vi "Lin Daten aufarbeiten.vi"(0 "Eingabetabelle":T4, 1 "Index (Seite)":i32, 3 "Stufen Tabelle":T3, 4 "Zeile":i32, 5 "Lin-Polynom":T5={"Messgerät"="", "Kalibrator (Gasteiler)"="", "Bearbeiter/in"="", "Komponente"="", "Zeitstempel"=timestamp(0 s since 1904-01-01), "F_max gefordert (%)"=0.0, "F_max in %"=0.0, "F_max in ppm"=0.0, "Vorschlag Ordnung"=0, "Polynom OK"=FALSE, "Polynomkoeff."=[], "Prüfgas Konzentration"=0.0, "Pfad EPA"="", "Pfad_LIN"="", "Gasnummer:"=0, "Komponentenauswahl"=[], "Verdünnungsgas"=0, "Zeitdauer Stufe"=0.0, "Anzahl Stufen"=0.0, "F_max in % EPA"=0.0, "F_max in ppm EPA"=0.0, "F_max in % LIN"=0.0, "F_max in ppm LIN"=0.0, "Punkte umkehren"=FALSE, "EPA Optionsfeld"=enum."Rohwert", "Autolin Hovacal"=enum."Optionsauswahl 2", "Spanfactors"=[], "Kalibrierauswahl"=0, "Conditions:"=0, "Gasflaschen Nr.:"="", "Bottle Accuracy"=0.0, "Konfig Gasflasche"=FALSE, "Gasflasche"=0, "HovaCAL Flow AutoLin"={"HovaCAL Flow Input Cluster"=0.0}, "MFC Output"={"Run"=FALSE}, "Gas Ablaufdatum"=timestamp(0 s since 1904-01-01), "Lin Modus"=0, "zusätzliche Zeitdauer Erster Punkt"=0.0, "Offsets"=[]} {"zusätzliche Zeitdauer Erster Punkt" format="%#_5g"; "Lin Modus" items=["Cal Gas to PNS", "Cal Gas to Samplepoint", "Measure"]; "Gas Ablaufdatum" format="%<%d.%m.%Y>T"; "HovaCAL Flow AutoLin"."HovaCAL Flow Input Cluster" format="%.2f"; "Gasflasche" items=["----"=10000, "IAG MG"=0, "IAG NH3 3000"=1, "IAG NH3 2000"=2, "IAG NH3 200"=3]; "Conditions:" items=["field", "laboratory"]; "Kalibrierauswahl" items=["Inaktiv", "Aktiv"]; "Anzahl Stufen" format="%#_5g"; "Zeitdauer Stufe" format="%#_5g"; "Verdünnungsgas" items=["N2", "O2"]; "Komponentenauswahl"."Konzentration" format="%#.6f"; "Gasnummer:" min=1 max=5; "Prüfgas Konzentration" format="%#.6f"; "Polynomkoeff." format="%#_18f"}, 6 "EGAK":string[](array[string]), 7 "error in (no error)":errorcluster caption="Fehler (Eingang, kein Fehler)", 8 "Polynom-Ordnung":i32, 9 "TabellenArray":string[][][](array[string]), 10 "Aktiv":T1, 12 "LINArray":bool[][](array[boolean]), 13 "Aktionen":T19, 14 "EPA Array":bool[][](array[boolean])) -> (16 "Aktiv EPA":T1, 17 "TabellenArray":string[][][](array[string]), 18 "Aktiv LIN":bool[](array[boolean]), 20 "Eingabetabelle":T4, 21 "Index (Seite) out":i32, 22 "Ergebnis Lin":string[][](array[string]), 23 "Stufen Tabelle":T3, 24 "EPA Auswertung":cluster{sgl[], sgl[], bool[]}, 25 "Lin-Polynom":T5={"Messgerät"="", "Kalibrator (Gasteiler)"="", "Bearbeiter/in"="", "Komponente"="", "Zeitstempel"=timestamp(0 s since 1904-01-01), "F_max gefordert (%)"=0.0, "F_max in %"=0.0, "F_max in ppm"=0.0, "Vorschlag Ordnung"=0, "Polynom OK"=FALSE, "Polynomkoeff."=[], "Prüfgas Konzentration"=0.0, "Pfad EPA"="", "Pfad_LIN"="", "Gasnummer:"=0, "Komponentenauswahl"=[], "Verdünnungsgas"=0, "Zeitdauer Stufe"=0.0, "Anzahl Stufen"=0.0, "F_max in % EPA"=0.0, "F_max in ppm EPA"=0.0, "F_max in % LIN"=0.0, "F_max in ppm LIN"=0.0, "Punkte umkehren"=FALSE, "EPA Optionsfeld"=enum."Rohwert", "Autolin Hovacal"=enum."Optionsauswahl 2", "Spanfactors"=[], "Kalibrierauswahl"=0, "Conditions:"=0, "Gasflaschen Nr.:"="", "Bottle Accuracy"=0.0, "Konfig Gasflasche"=FALSE, "Gasflasche"=0, "HovaCAL Flow AutoLin"={"HovaCAL Flow Input Cluster"=0.0}, "MFC Output"={"Run"=FALSE}, "Gas Ablaufdatum"=timestamp(0 s since 1904-01-01), "Lin Modus"=0, "zusätzliche Zeitdauer Erster Punkt"=0.0, "Offsets"=[]} {"zusätzliche Zeitdauer Erster Punkt" format="%#_5g"; "Lin Modus" items=["Cal Gas to PNS", "Cal Gas to Samplepoint", "Measure"]; "Gas Ablaufdatum" format="%<%d.%m.%Y>T"; "HovaCAL Flow AutoLin"."HovaCAL Flow Input Cluster" format="%.2f"; "Gasflasche" items=["----"=10000, "IAG MG"=0, "IAG NH3 3000"=1, "IAG NH3 2000"=2, "IAG NH3 200"=3]; "Conditions:" items=["field", "laboratory"]; "Kalibrierauswahl" items=["Inaktiv", "Aktiv"]; "Anzahl Stufen" format="%#_5g"; "Zeitdauer Stufe" format="%#_5g"; "Verdünnungsgas" items=["N2", "O2"]; "Komponentenauswahl"."Konzentration" format="%#.6f"; "Gasnummer:" min=1 max=5; "Prüfgas Konzentration" format="%#.6f"; "Polynomkoeff." format="%#_18f"}, 26 "EKAG":string[](array[string]), 27 "error out":errorcluster caption="Fehler (Ausgang)")   [LabVIEW 2020, in "Linearisierung v2.lvlib"]
uses:
  Linearisierung v2.lvlib
  Aktion Lin Daten aufarbeiten.ctl
  Lin-Polynom Daten.ctl
  KomponentenArray.ctl
  Visualisierungs Elemente/Auswahlfeld.ctl
  Visualisierungs Elemente/Zahlen-Eingabefeld.ctl
  EPA Optionsfeld.ctl
  Gasteiler/HovaCal/AutoLin Hovacal.ctl
  Kalibrieroption.ctl
  EPA1065-307/Condition.ctl
  Seiten/System Einstellungen V2/Konfig Gasflasche.ctl
  Seiten/System Einstellungen V2/Gasflasche Auswahl.ctl
  Gasteiler/HovaCAL_Interface/Controls/Flow Einstellung.ctl
  Gasteiler/HovaCAL_Interface/Controls/Pump state.ctl
  Seiten/CalGas Aufschaltung/Lin Modus.ctl
  Eingabetabelle.ctl
  Gasteiler/Stufen Tabelle.ctl
  AktivArray.ctl
  AktivButton.ctl
  Sprachverwaltung/FGV Aktion Tabelle zerlegen.ctl
  Allgemein/allgemeine Sub-VIs.lvlib
  EPA1065-307/Linearity verification 1065-307.lvlib
  Sprachverwaltung/Sprachverwaltung.lvlib
  Gasteiler/Gasteiler.lvlib
  Gasteiler/HovaCal/HovaCal.lvlib
  Seiten/System Einstellungen V2/System Einstellungen V2.lvlib
  Gasteiler/HovaCAL_Interface/Controls/Controls.lvlib
  Seiten/CalGas Aufschaltung/CalGas Aufschaltung.lvlib
panel:
  # "Tabelle:\n0.....Sollwert\n1.....Istwert\n2.....Rohwert\n3.....linearisiert\n4.....abs.Fehler ppm\n5.....Fehler in %\n6.....Deviation\n7.....Temp.Messzelle\n8.....Druck Messzelle\n9.....abs.Fehler ppm linearisiert\n10....Fehler in % linearisiert\n11....abs.Fehler ppm EPA\n12....Fehler in % EPA\n13....abs.Fehler ppm Rohwert\n14....Fehler in % Rohwert"
  # "%"
  # "%"
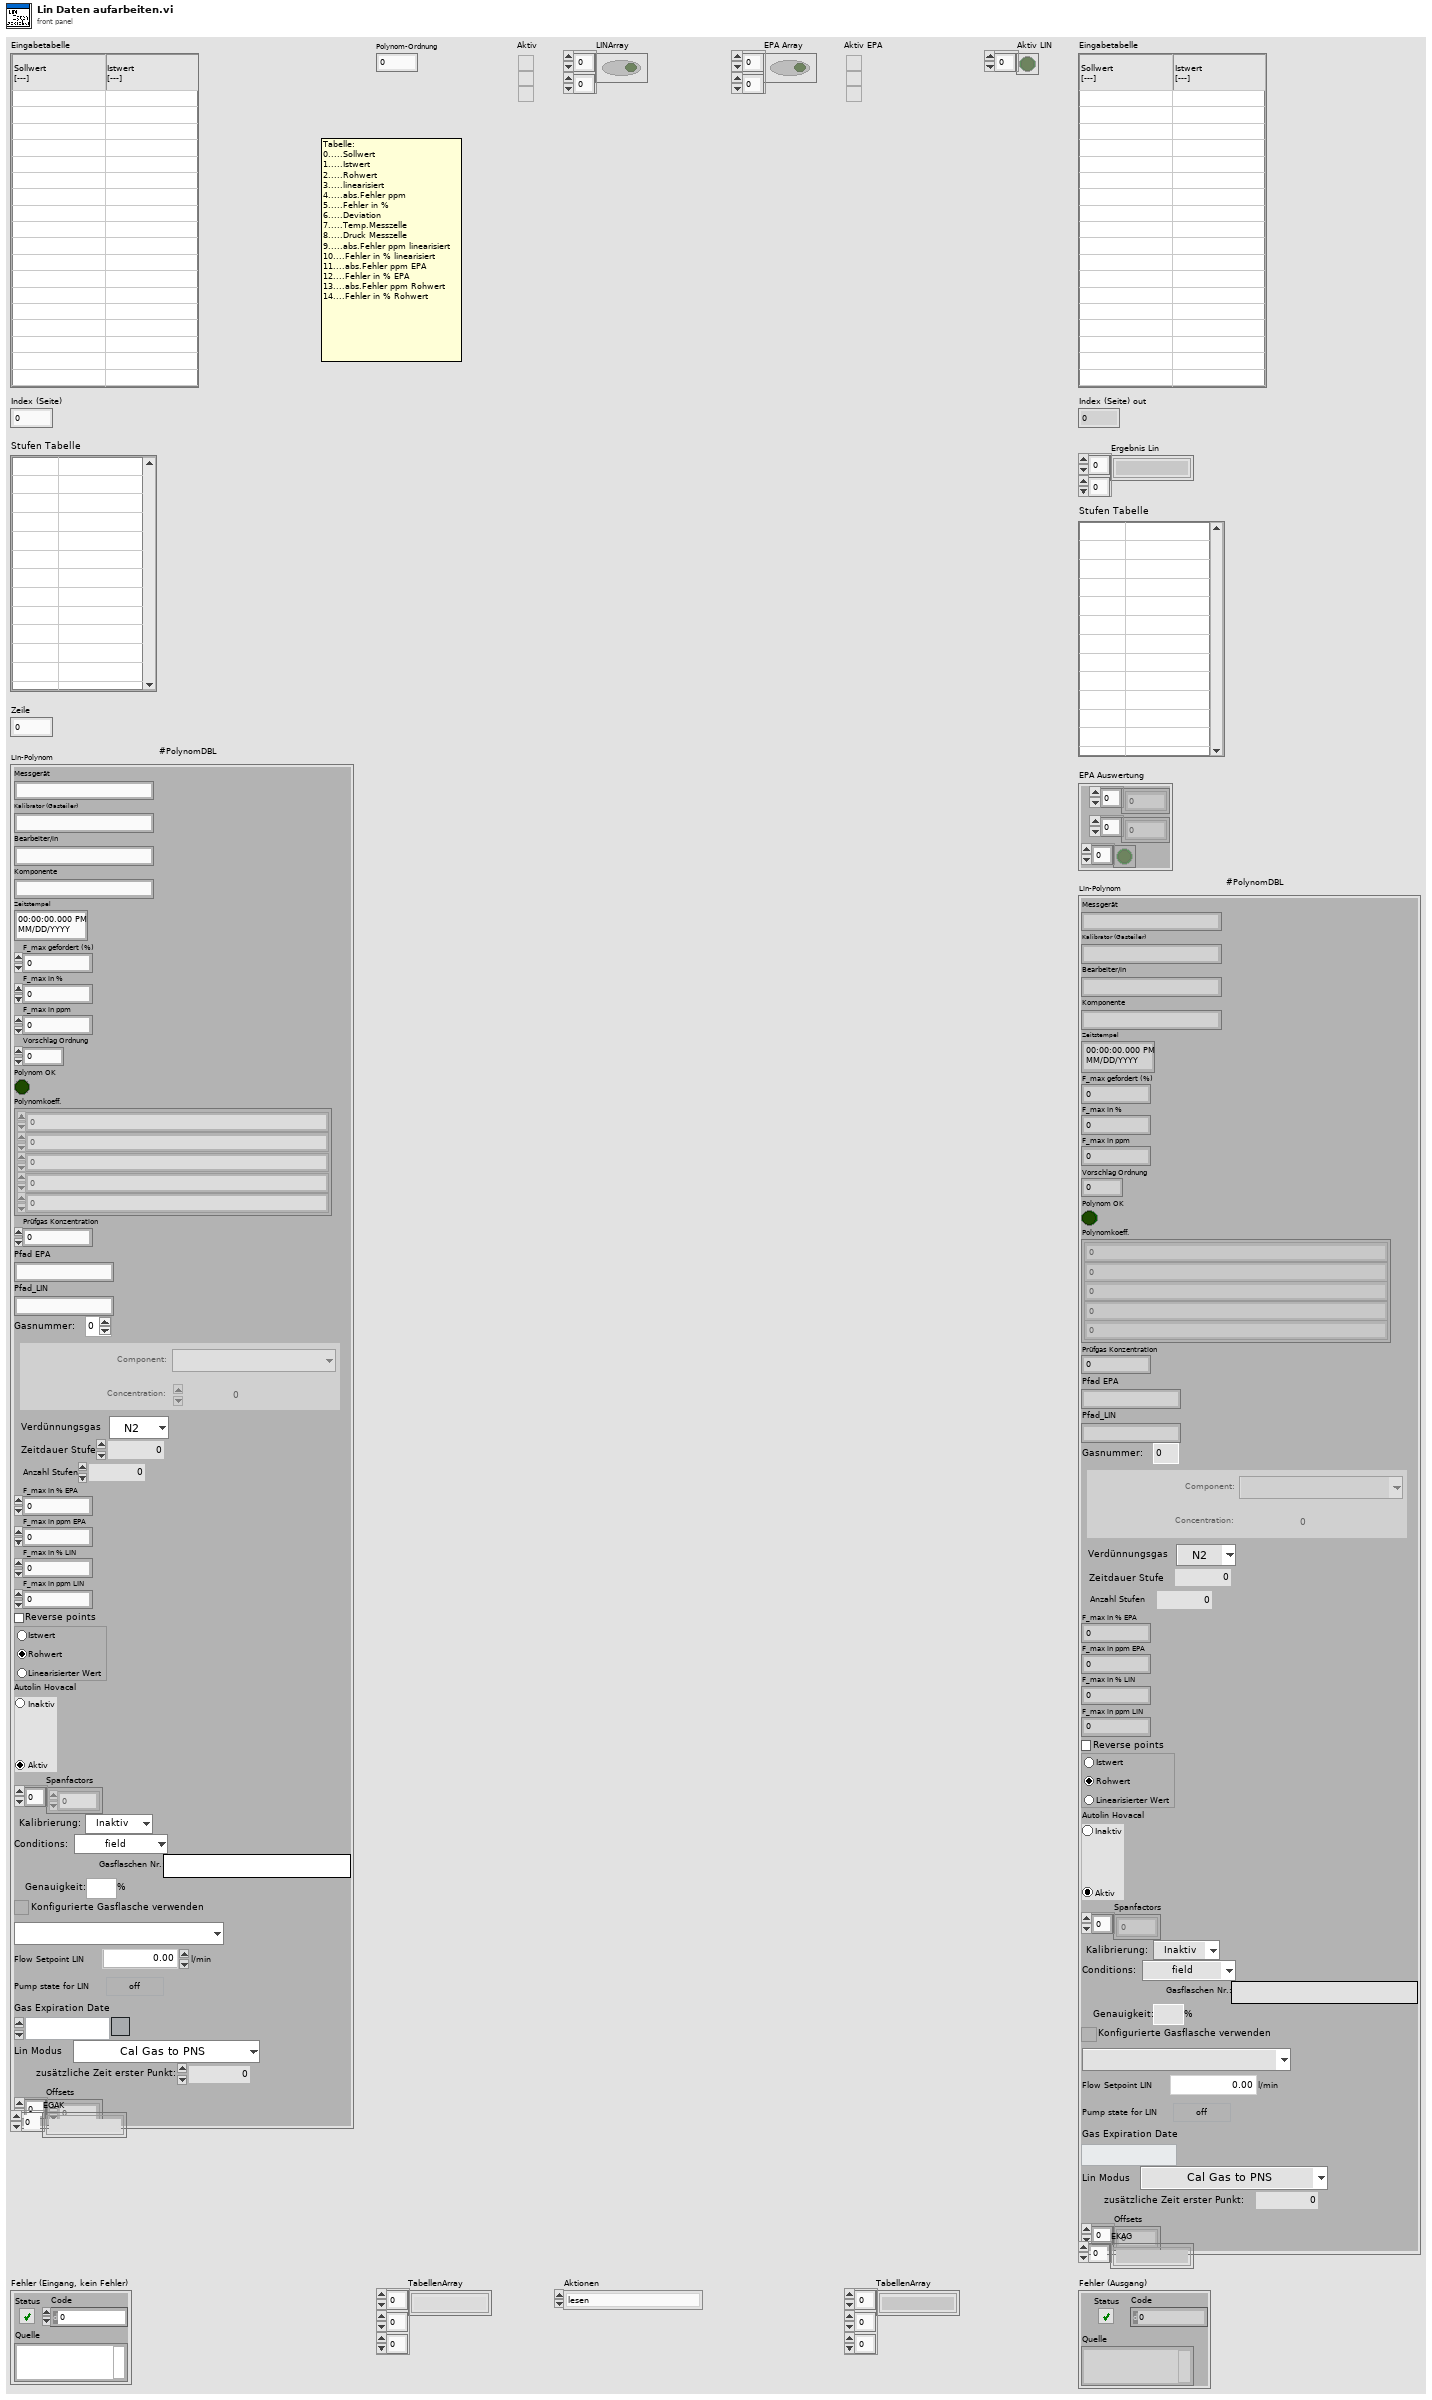
[diagram p1: front panel]
types:
  T1 = typedef "Linearisierung v2.lvlib/AktivArray.ctl" = T2[]
  T2 = typedef "Linearisierung v2.lvlib/AktivButton.ctl" = bool
  T3 = typedef "Linearisierung v2.lvlib/Gasteiler.lvlib/Stufen Tabelle.ctl" = string[][]
  T4 = typedef "Linearisierung v2.lvlib/Eingabetabelle.ctl" = string[][]
  T5 = typedef "Linearisierung v2.lvlib/Lin-Polynom Daten.ctl" = cluster{"Messgerät":string, "Kalibrator (Gasteiler)":string, "Bearbeiter/in":string, "Komponente":string, "Zeitstempel":timestamp, "F_max gefordert (%)":sgl, "F_max in %":sgl, "F_max in ppm":sgl, "Vorschlag Ordnung":i32, "Polynom OK":bool, "Polynomkoeff.":dbl[], "Prüfgas Konzentration":dbl, "Pfad EPA":string, "Pfad_LIN":string, "Gasnummer:":u8, "Komponentenauswahl":T6, "Verdünnungsgas":T8, "Zeitdauer Stufe":T9, "Anzahl Stufen":T9, "F_max in % EPA":sgl, "F_max in ppm EPA":sgl, "F_max in % LIN":sgl, "F_max in ppm LIN":sgl, "Punkte umkehren":bool, "EPA Optionsfeld":T10, "Autolin Hovacal":T11, "Spanfactors":sgl[], "Kalibrierauswahl":T12, "Conditions:":T13, "Gasflaschen Nr.:":string, "Bottle Accuracy":dbl, "Konfig Gasflasche":T14, "Gasflasche":T15, "HovaCAL Flow AutoLin":T16, "MFC Output":T17, "Gas Ablaufdatum":timestamp, "Lin Modus":T18, "zusätzliche Zeitdauer Erster Punkt":sgl, "Offsets":sgl[]}
  T6 = typedef "Linearisierung v2.lvlib/KomponentenArray.ctl" = cluster{"Komponente:":T7, "Konzentration":dbl}[]
  T7 = typedef "Auswahlfeld.ctl" = u16
  T8 = typedef "Linearisierung v2.lvlib/Gasteiler.lvlib/Prüfgas in.ctl" = u16
  T9 = typedef "Zahlen-Eingabefeld.ctl" = sgl
  T10 = typedef "Linearisierung v2.lvlib/EPA Optionsfeld.ctl" = enum32{"Istwert", "Rohwert", "Linearisierter Wert"}
  T11 = typedef "Linearisierung v2.lvlib/Gasteiler.lvlib/HovaCal.lvlib/AutoLin Hovacal.ctl" = enum32{"Keine Auswahl", "Optionsauswahl 1", "Optionsauswahl 2"}
  T12 = typedef "Linearisierung v2.lvlib/Kalibrieroption.ctl" = u16
  T13 = typedef "Linearisierung v2.lvlib/Linearity verification 1065-307.lvlib/Condition.ctl" = u16
  T14 = typedef "System Einstellungen V2.lvlib/Konfig Gasflasche.ctl" = bool
  T15 = typedef "System Einstellungen V2.lvlib/Gasflasche Auswahl.ctl" = u16
  T16 = typedef "Linearisierung v2.lvlib/Gasteiler.lvlib/HovaCAL_Interface.lvlib/Controls.lvlib/Flow Einstellung.ctl" = cluster{"HovaCAL Flow Input Cluster":dbl}
  T17 = typedef "Linearisierung v2.lvlib/Gasteiler.lvlib/HovaCAL_Interface.lvlib/Controls.lvlib/Pump state.ctl" = cluster{"Run":bool}
  T18 = typedef "CalGas Aufschaltung.lvlib/Lin Modus.ctl" = u16
  T19 = typedef "Linearisierung v2.lvlib/Aktion Lin Daten aufarbeiten.ctl" = enum16{"lesen", "Protkolldaten", "speichern", "laden", "EPA auswerten", "Tabelle schreiben", "Lin auswerten", "Tab init", "Stufentabelle", "EPA aktiviert", "Nachbehandlung laden", "Tabelle löschen", "Istwerte löschen", "Zeile löschen", "Zeile einfügen", "LIN aktiviert", "LIN/EPA aktiv laden", "EGAK Tab", "LIN übernehmen", "Tab init ohne Stufen"}
  T20 = typedef "Sprachverwaltung.lvlib/FGV Aktion Tabelle zerlegen.ctl" = enum16{"laden", "vereinzeln", "speichern"}
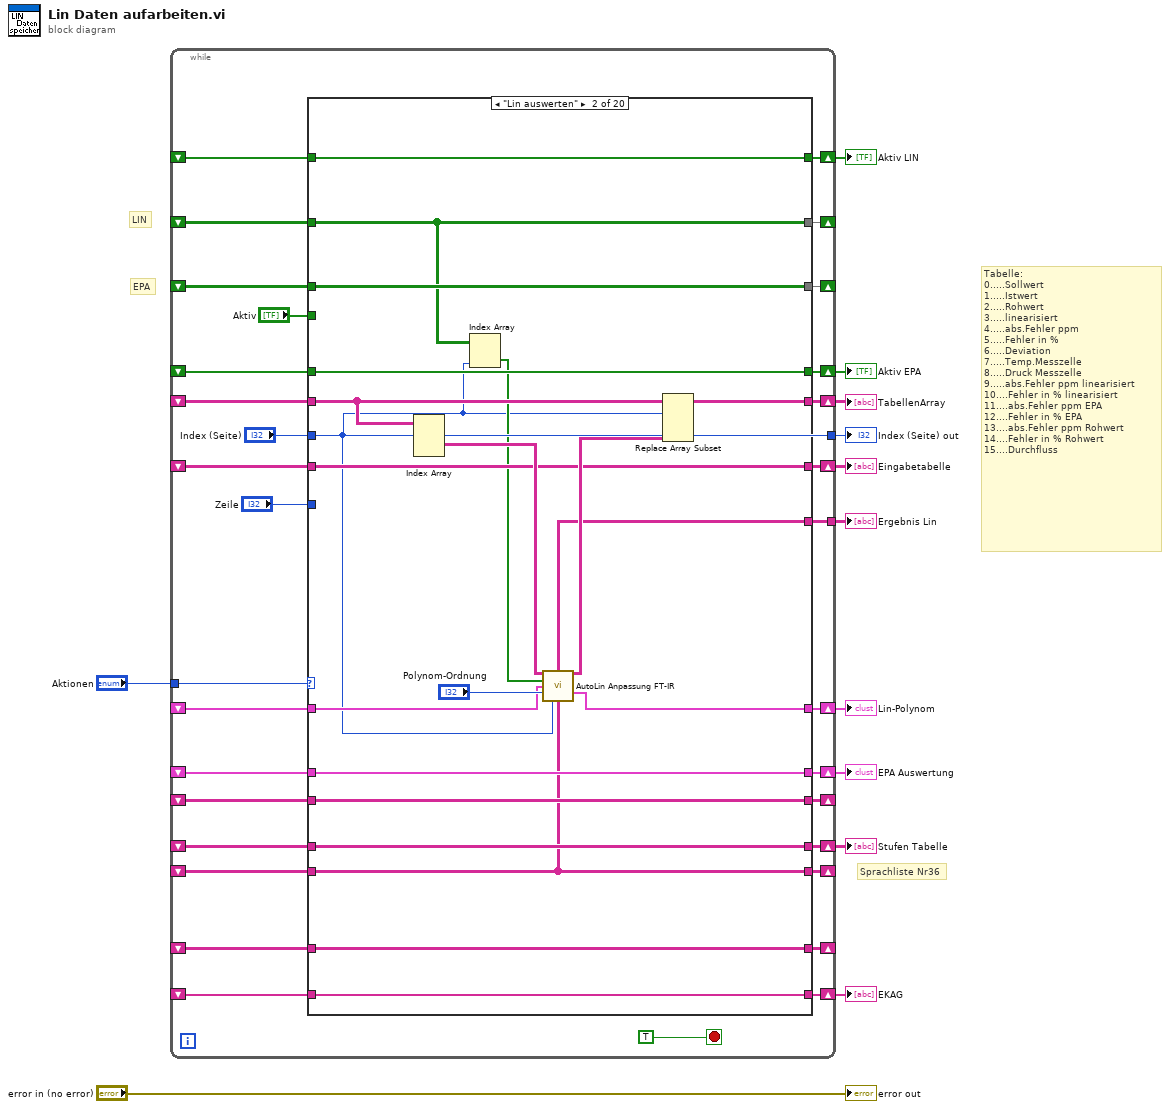
[diagram p0: block diagram]
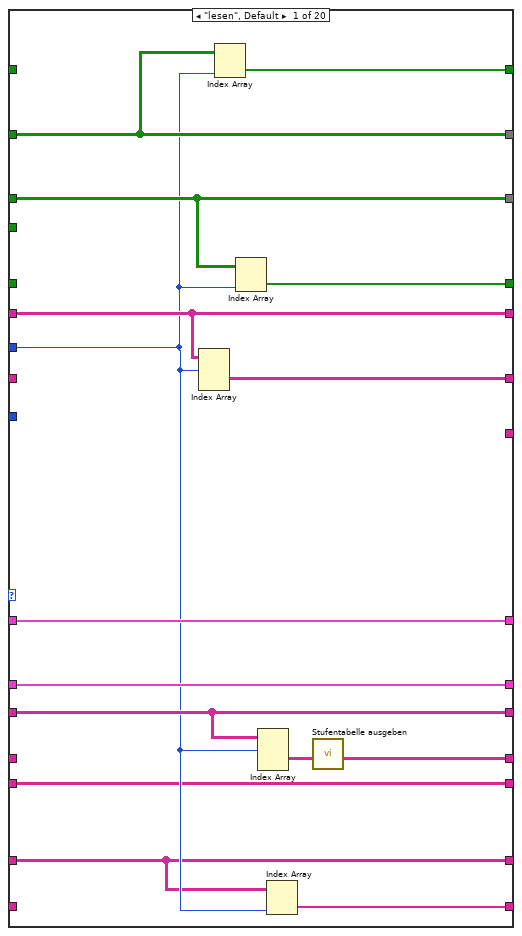
[diagram p2: hidden frame]
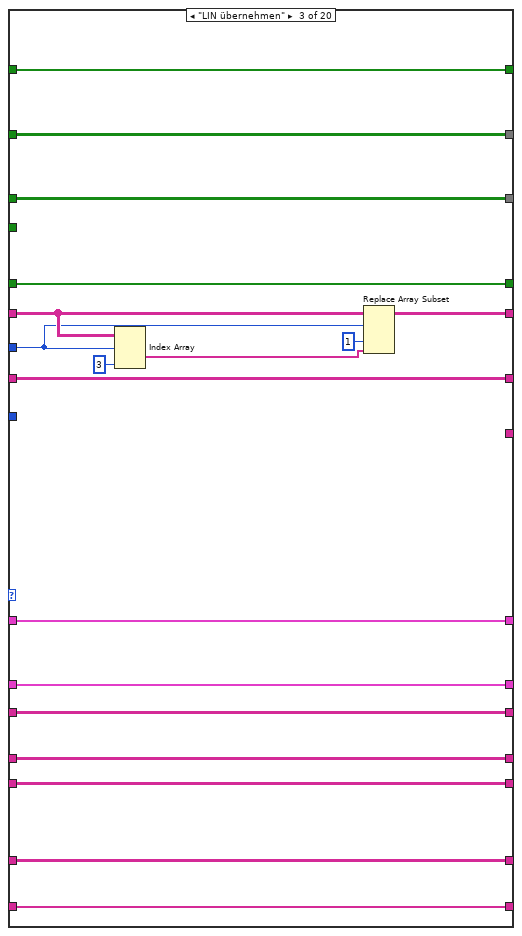
[diagram p3: hidden frame]
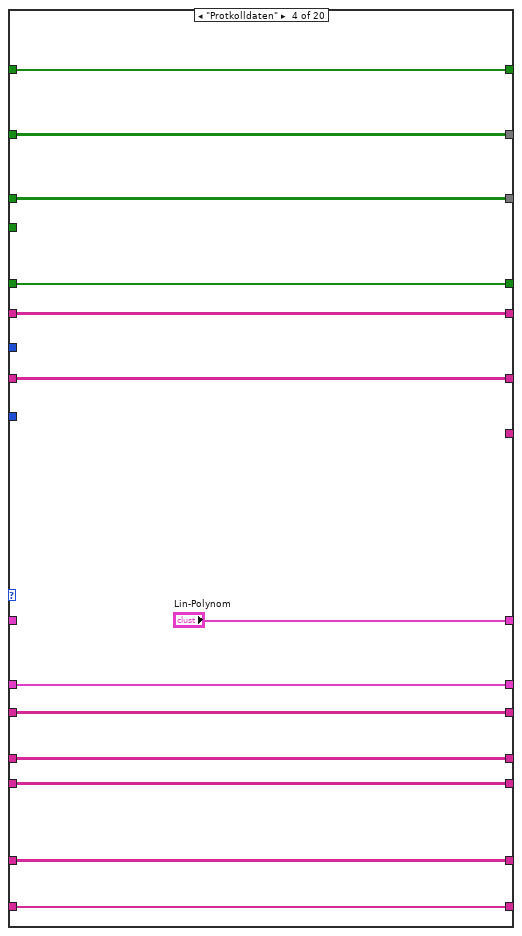
[diagram p4: hidden frame]
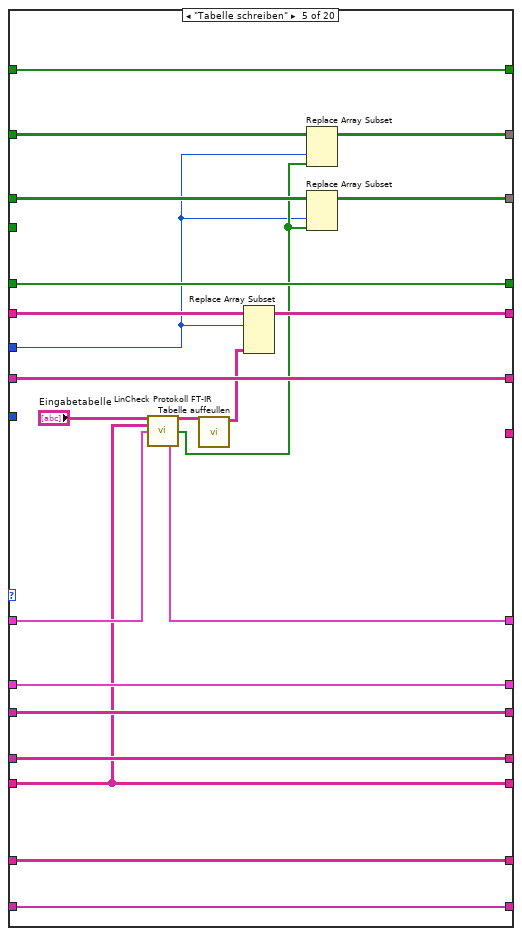
[diagram p5: hidden frame]
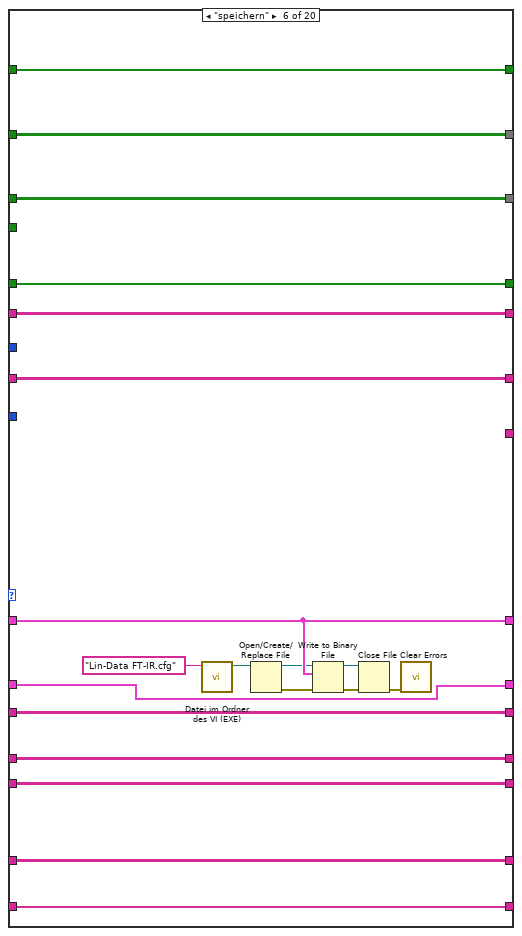
[diagram p6: hidden frame]
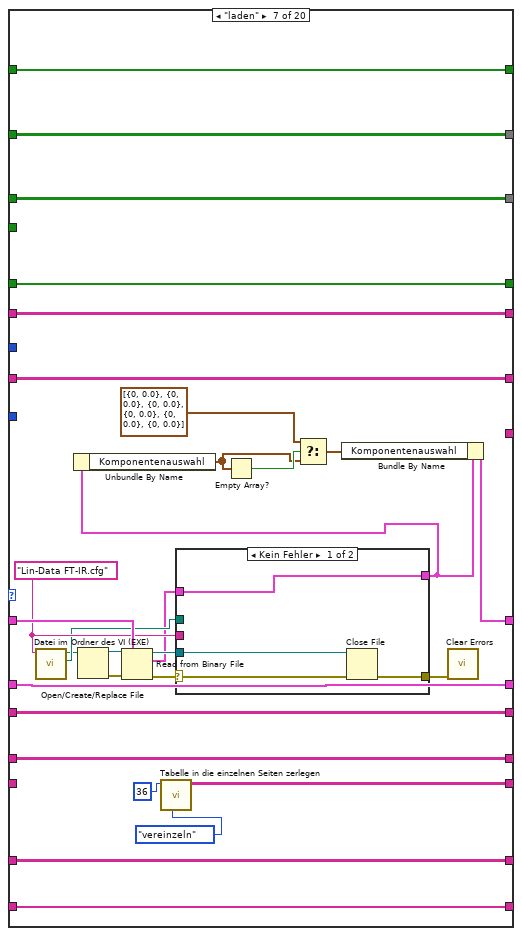
[diagram p7: hidden frame]
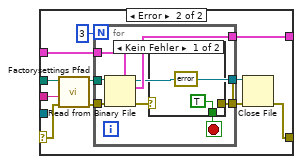
[diagram p8: hidden frame]
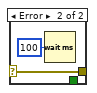
[diagram p9: hidden frame]
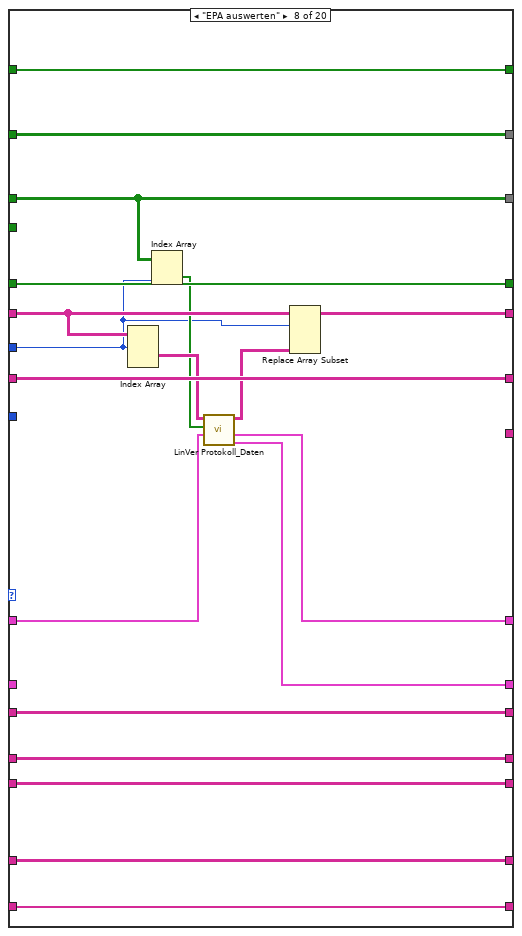
[diagram p10: hidden frame]
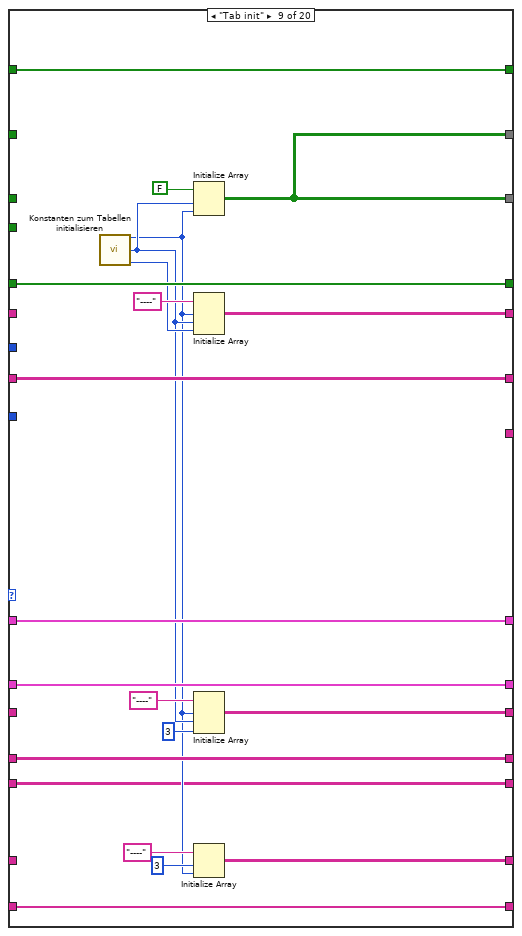
[diagram p11: hidden frame]
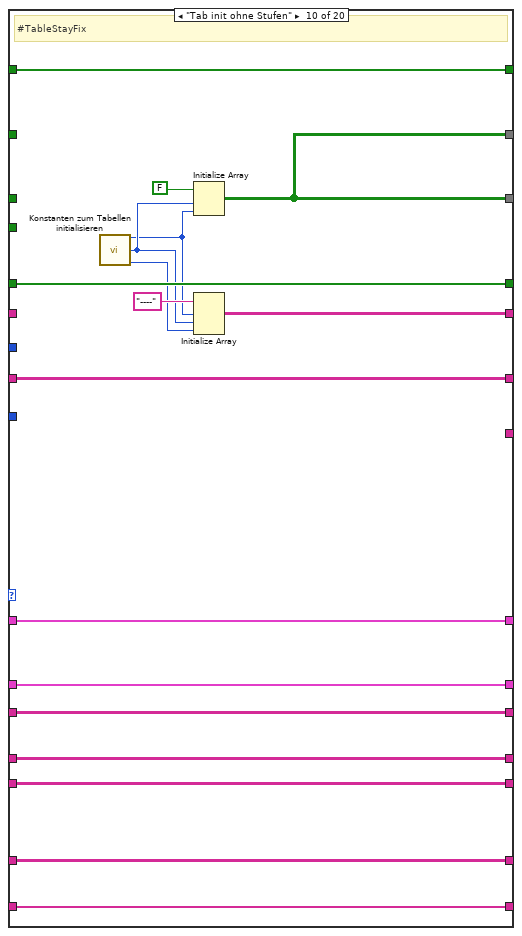
[diagram p12: hidden frame]
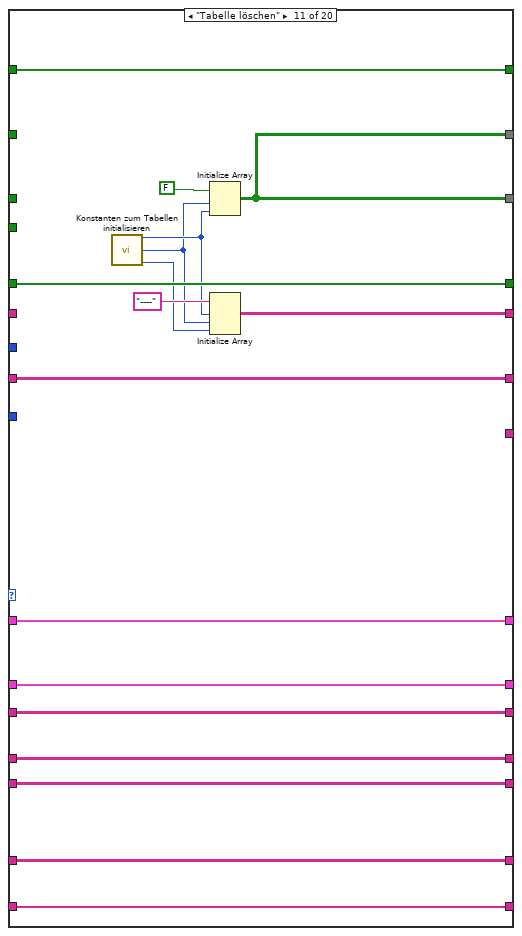
[diagram p13: hidden frame]
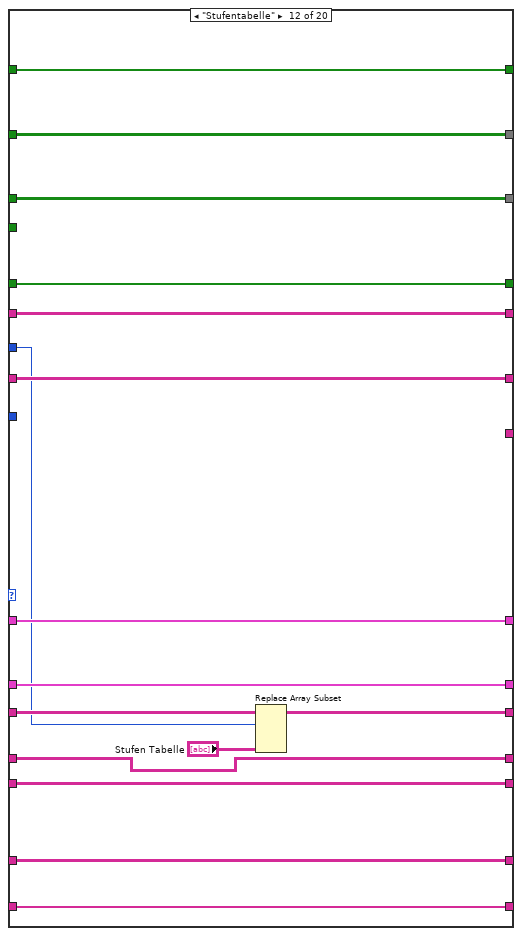
[diagram p14: hidden frame]
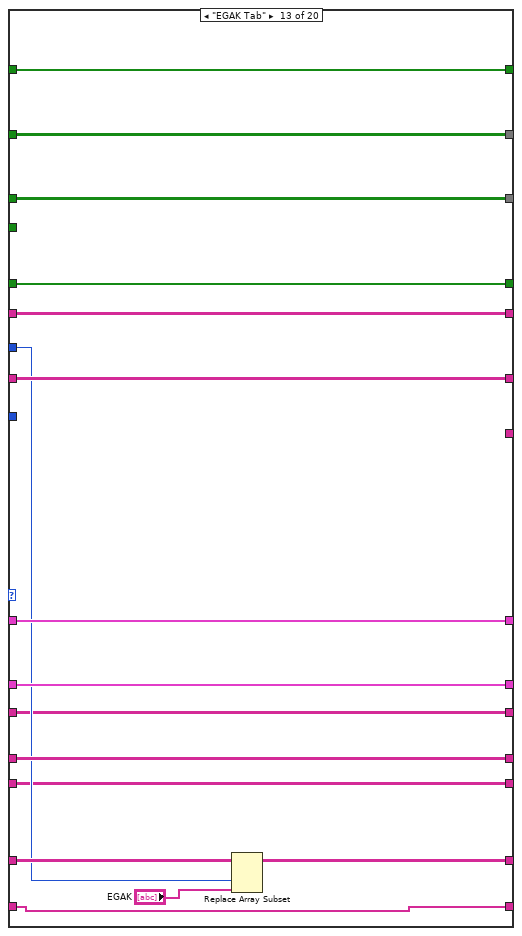
[diagram p15: hidden frame]
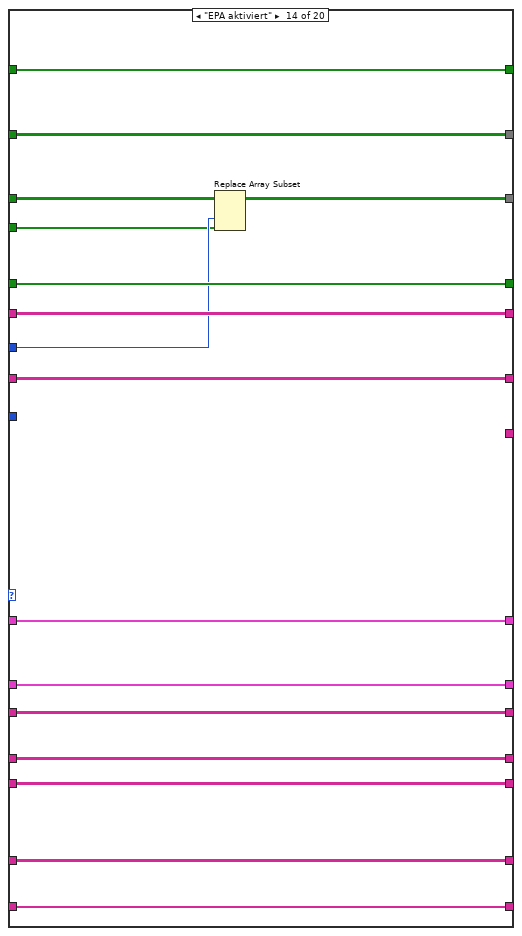
[diagram p16: hidden frame]
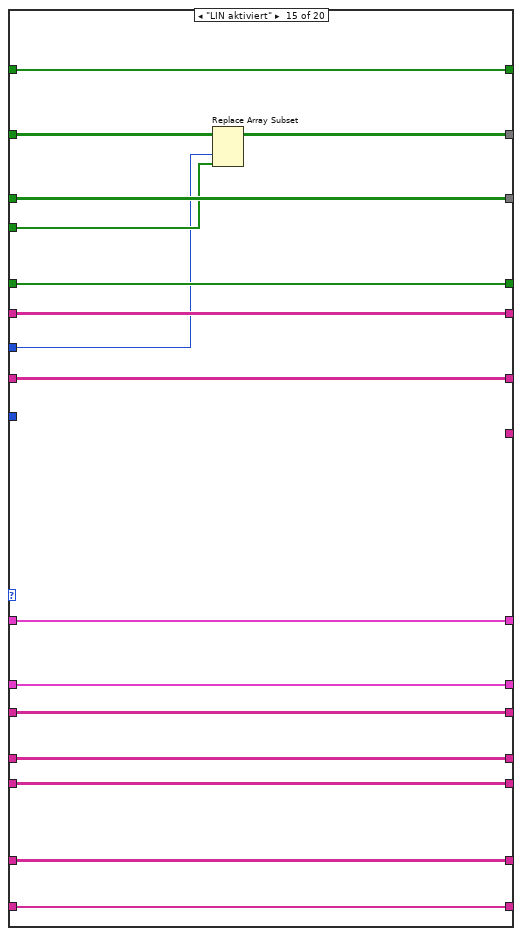
[diagram p17: hidden frame]
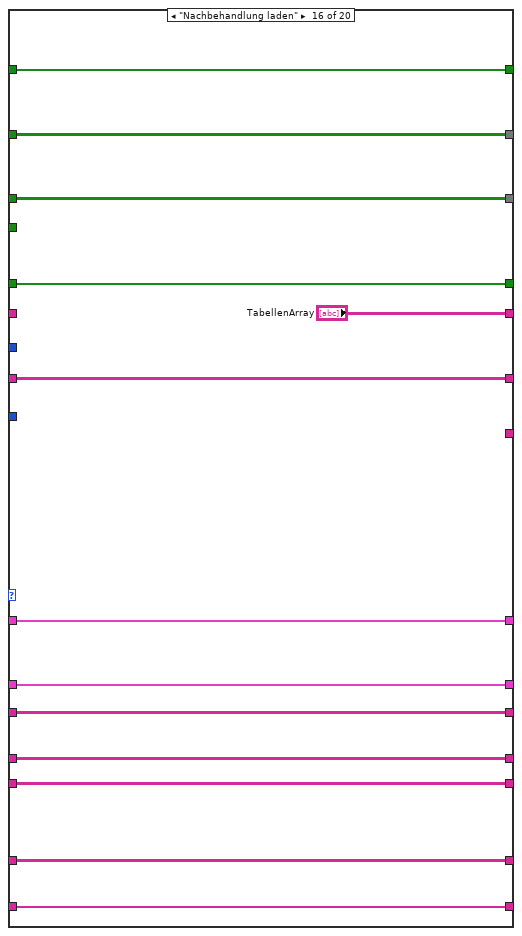
[diagram p18: hidden frame]
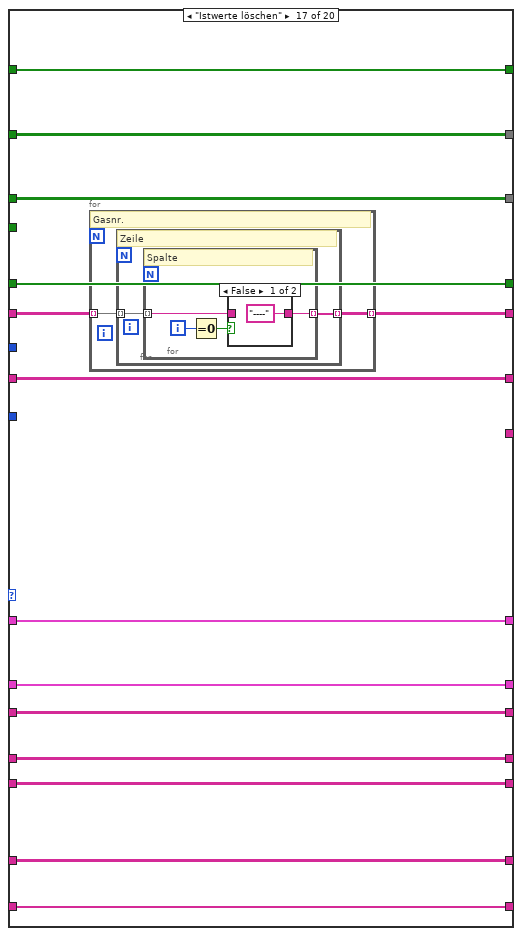
[diagram p19: hidden frame]
diagram:
  # "Sprachliste Nr36"
  # "LIN"
  # "EPA"
  # "Tabelle:\n0.....Sollwert\n1.....Istwert\n2.....Rohwert\n3.....linearisiert\n4.....abs.Fehler ppm\n5.....Fehler in %\n6.....Deviation\n7.....Temp.Messzelle\n8.....Druck Messzelle\n9.....abs.Fehler ppm linearisiert\n10....Fehler in % linearisiert\n11....abs.Fehler ppm EPA\n12....Fehler in % EPA\n13....abs.Fehler ppm Rohwert\n14....Fehler in % Rohwert\n15....Durchfluss"
  n1 = while {
    tunnel: "Aktionen" -> [w43]
    shift-right: [w42] -> w6
    shift-left: _ -> [w41]
    shift-right: [w40] -> w11
    shift-left: _ -> [w39]
    shift-right: [w38] -> w7
    shift-left: _ -> [w37]
    shift-right: [w36] -> w10
    shift-left: _ -> [w35]
    shift-right: [w34] -> _
    shift-left: _ -> [w33]
    shift-right: [w32] -> w9
    shift-left: _ -> [w31]
    shift-right: [w30] -> w8
    shift-left: _ -> [w29]
    shift-right: [w28] -> _
    shift-left: _ -> [w27]
    shift-right: [w25] -> _
    shift-left: _ -> [w24]
    shift-right: [w22] -> w5
    shift-left: _ -> [w21]
    shift-right: [w20] -> _
    shift-left: _ -> [w19]
    shift-right: [w18] -> w4
    shift-left: _ -> [w17]
    tunnel: [w16] -> w3
    tunnel: ["Index (Seite)"] -> w2
    shift-right: [w14] -> _
    shift-left: _ -> [w13]
    stop <- TRUE stop-if-true
    n2 = case shown="\"Lin auswerten\"" w43 {
      tunnel: [w59 w69 w85 "Lin-Polynom" w120 w152 w159 w222 w249 w266 w283 w297 w313 w332 w348 w361 w375 w406 w441 w467] -> w42
      tunnel: w41 -> [w59 w70 w85 _ w132 w152 w183 w227 w249 w266 w283 w297 w313 w332 w348 w361 w375 w406 w441 w467]
      tunnel: [w57 w75 w96 w110 w129 w151 w182 w229 w250 w267 w284 w300 w316 w331 w347 w360 w374 w405 w440 w466] -> w40
      tunnel: w39 -> [_ w75 w96 w110 w129 w151 w182 w229 w250 w267 w284 w300 w316 w331 w347 w360 w374 w405 w440 w466]
      tunnel: [w58 w77 w97 w109 w130 w150 w181 w225 w247 w264 w281 w299 w315 w330 w346 "TabellenArray" w367 w399 w434 w465] -> w38
      tunnel: w37 -> [w58 w79 w98 w109 w131 w150 w181 w226 _ _ _ w299 w315 w330 w346 _ w368 w400 w435 w465]
      tunnel: "Index (Seite)" -> [w48 w61 w86 _ w116 _ _ w216 _ _ _ w294 w304 w323 w339 _ _ _ _ _]
      tunnel: [w56 w74 w95 w108 w128 w149 w180 w223 w246 w263 w280 w298 w314 w329 w345 w359 w373 w404 w439 w464] -> w36
      tunnel: w35 -> [w56 w74 w95 w108 w128 w149 w180 _ w246 w263 w280 w298 w314 w329 w345 w359 w373 w404 w439 w464]
      tunnel: [w55 w73 w94 w107 w127 w148 w179 w221 w243 w253 w276 w295 w303 w328 w344 w358 w372 w403 w438 w463] -> w34
      tunnel: w33 -> [w55 w73 w94 w107 w127 w148 w179 w221 _ w253 w276 w296 w303 w328 w344 w358 w372 w403 w438 w463]
      tunnel: [w51 w72 w93 w106 w126 w147 w178 w220 w242 w262 w279 w292 w312 w327 w343 w357 w371 w402 w437 w462] -> w32
      tunnel: w31 -> [_ w72 w93 w106 w126 w147 w178 w220 w242 w262 w279 w292 w312 w327 w343 w357 w371 w402 w437 w462]
      tunnel: [w53 w71 w92 w105 w121 w146 w177 w219 w241 w261 w278 w291 w311 w326 w342 w356 w370 w401 w436 w461] -> w30
      tunnel: w29 -> [_ w71 w92 w105 w121 w146 w177 w219 w241 w261 w278 w291 w311 w326 w342 w356 w370 w401 w436 w461]
      tunnel: [w54 w68 w91 w104 w122 w145 w176 w218 w239 w259 w275 w290 w310 w324 w341 w352 w369 w395 w430 "EPA Array"] -> w28
      tunnel: w27 -> [w54 w68 w91 w104 w123 w145 w176 w218 _ _ _ w290 w310 w325 w341 w352 w369 w397 w432 _]
      tunnel: "Zeile" -> [_ _ _ _ _ _ _ _ _ _ _ _ _ _ _ _ _ w390 w425 _]
      tunnel: [w49 w65 w89 w102 w117 w144 w174 w215 w239 w259 w275 w289 w309 w321 w337 w353 w365 w391 w426 "LINArray"] -> w25
      tunnel: w24 -> [w49 w65 w89 w102 w118 w144 w174 w215 _ _ _ w289 w309 w321 w338 w353 w365 w392 w427 _]
      tunnel: "Aktiv" -> [_ _ _ _ _ _ _ _ _ _ _ _ _ w322 w340 _ _ _ _ _]
      tunnel: [w50 w66 w90 w103 w115 w143 w175 w214 w238 w258 w274 w288 w308 w320 w336 w354 w366 w389 w424 w460] -> w22
      tunnel: w21 -> [_ w66 w90 w103 w115 w143 w175 w214 w238 w258 w274 w288 w308 w320 w336 w354 w366 w389 w424 w460]
      tunnel: [w47 w64 w88 w101 w114 w142 w173 w213 w235 w252 w273 w287 w306 w319 w335 w351 w364 w388 w423 w457] -> w20
      tunnel: w19 -> [w47 w64 w88 w101 w114 w142 w173 w213 _ w252 w273 w287 w307 w319 w335 w351 w364 w388 w423 w457]
      tunnel: [w46 w63 w87 w100 w113 w141 w172 w212 w234 w257 w272 w286 w302 w318 w334 w350 w363 w387 w422 w456] -> w18
      tunnel: w17 -> [_ w63 w87 w100 w113 w141 w172 w212 w234 w257 w272 w286 w302 w318 w334 w350 w363 w387 w422 w456]
      tunnel: [_ w62 _ _ _ _ _ _ _ _ _ _ _ _ _ _ _ _ _ _] -> w16
      tunnel: [w45 w60 w81 w99 w112 w134 w154 w211 w230 w251 w268 w285 w301 w317 w333 w349 w362 w386 w421 w455] -> w14
      tunnel: w13 -> [w45 w60 w81 w99 w112 w134 _ w211 w230 w251 w268 w285 w301 w317 w333 w349 w362 w386 w421 w455]
      frame "lesen", Default {
        n3 = Index Array(array=w58, index (dim 0)=w48) -> (element=w57:string[][])  [unwired: 2 in]
        n4 = Index Array(array=w49, index (col)=w48) -> (element=w50:bool[])  [unwired: 1 in]
        n5 = Index Array(array=w54, index (col)=w48) -> (element=w53:bool[])  [unwired: 1 in]
        n6 = Index Array(array=w55, index (dim 0)=w48) -> (element=w52:string[][])  [unwired: 2 in]
        n7 = Index Array(array=w47, index (col)=w48) -> (element=w46:string[])  [unwired: 1 in]
        n8 = call "Stufentabelle ausgeben.vi"("Neue Tabelle"=w52) -> ("Tabelle"=w51:string[][])  [unwired: 10 in]
      }
      frame "Lin auswerten" {
        n9 = Index Array(array=w79, index (dim 0)=w61) -> (element=w78:string[][])  [unwired: 2 in]
        n10 = Index Array(array=w65, index (col)=w61) -> (element=w67:bool[])  [unwired: 1 in]
        n11 = call "AutoLin Anpassung FT-IR.vi"("Eingabetabelle"=w78, "Aktiv"=w67, "Lin-Polynom"=w70, "Polynom-Ordnung"="Polynom-Ordnung", "Index (Seite)"=w61, "Sprachliste"=w60) -> ("Ergebnis Lin"=w62:string[][], "Tabelle"=w76:T4, "Lin-Polynom"=w69:T5)  [unwired: 6 in, 1 out]
        n12 = Replace Array Subset(array=w79, new element=w76, index (dim 0)=w61) -> (w77:string[][][])  [unwired: 2 in]
      }
      frame "LIN übernehmen" {
        n13 = Index Array(array=w98, index (dim 0)=w86, index (dim 2)=3 ("Deaktivierter Index (Spalte)")) -> (element=w82:string[])  [unwired: 1 in]
        n14 = Replace Array Subset(array=w98, new element=w82, index (dim 0)=w86, index (dim 2)=1 ("Deaktivierter Index (Spalte)")) -> (w97:string[][][])  [unwired: 1 in]
      }
      frame "Protkolldaten" {
      }
      frame "Tabelle schreiben" {
        n15 = call "LinCheck Protokoll FT-IR.vi"("Eingabetabelle"="Eingabetabelle", "Sprachliste"=w112, "Lin-Polynom Daten"=w132) -> ("Eingabetabelle erweitert"=w125:string[][], "Aktiv"=w119:T1, "Lin-Polynom Daten"=w120:T5)  [unwired: 7 in, 3 out]
        n16 = call "Tabelle auffeullen.vi"("Neue Tabelle"=w125) -> ("Tabelle"=w124:string[][])  [unwired: 10 in]
        n17 = Replace Array Subset(array=w131, new element=w124, index (dim 0)=w116) -> (w130:string[][][])  [unwired: 2 in]
        n18 = Replace Array Subset(array=w118, new element=w119, index (col)=w116) -> (w117:bool[][])  [unwired: 1 in]
        n19 = Replace Array Subset(array=w123, new element=w119, index (col)=w116) -> (w122:bool[][])  [unwired: 1 in]
      }
      frame "speichern" {
        n20 = call "Datei im Ordner des VI (EXE).vi"("Dateiname"="Lin-Data FT-IR.cfg") -> ("Dateipfad im Ordner des Haupt-VIs"=w140:path)  [unwired: 8 in, 2 out]
        n21 = Open/Create/Replace File(file path (use dialog)=w140) -> (refnum out=w136:refnum<file>, error out=w139:errorcluster)  [unwired: 5 in, 1 out]
        n22 = Write to Binary File(file (use dialog)=w136, data=w152, error in=w139) -> (refnum out=w135:refnum<file>, error out=w137:errorcluster)  [unwired: 4 out]
        n23 = Close File(refnum=w135, error in=w137) -> (error out=w138:errorcluster)  [unwired: 1 out]
        n24 = call <vilib>:"Clear Errors.vi"("error in (no error)"=w138) -> ()  [unwired: 5 in, 2 out]
      }
      frame "laden" {
        w169 = "Lin-Data FT-IR.cfg" ("Dateiname")
        n25 = call "Datei im Ordner des VI (EXE).vi"("Dateiname"=w169) -> ("Ordner des Haupt-VIs"=w168:path, "Dateipfad im Ordner des Haupt-VIs"=w165:path)  [unwired: 8 in, 1 out]
        n26 = Open/Create/Replace File(file path (use dialog)=w165) -> (refnum out=w164:refnum<file>, error out=w163:errorcluster)  [unwired: 5 in, 1 out]
        n27 = Read from Binary File(5:w183, 8:w163, 11:w164) -> (0:w171:errorcluster, 2:w166:T5, 3:w167:refnum<file>)  [unwired: 4 out]
        n28 = call "Tabelle in die einzelnen Seiten zerlegen.vi"("Aktion"=FGV_Aktion_Tabelle_zerlegen."vereinzeln", "Index (Seite)"=36) -> ("Sprachliste"=w154:string[][])  [unwired: 7 in, 2 out]
        n29 = case shown="Kein Fehler" w171 {
          selector: w171 -> [w186 w190]
          tunnel: w168 -> [_ w191]
          tunnel: w166 -> [w187 w189]
          tunnel: [w187 w197] -> w158
          tunnel: [w184 w195] -> w170
          tunnel: w167 -> [w185 _]
          tunnel: w169 -> [_ w188]
          frame No Error {
            n30 = Close File(refnum=w185, error in=w186) -> (error out=w184:errorcluster)  [unwired: 1 out]
          }
          frame Error {
            n31 = call "Factorysettings Pfad.vi"("error in (no error)"=w190, "Dateiname"=w188, "Ordner des Haupt-VIs"=w191) -> ("error out"=w192:errorcluster, "Pfad Factorysettings"=w193:path)  [unwired: 7 in]
            n32 = for {
              N: 3 -> [_]
              tunnel: w192 -> [w204]
              tunnel: w193 -> [w203]
              tunnel: [w202] -> w197
              tunnel: [w201] -> w196
              tunnel: [w200] -> w194
              tunnel: w189 -> [w199]
              stop <- w205 stop-if-true
              n33 = Read from Binary File(5:w199, 8:w204, 11:w203) -> (0:w206:errorcluster, 2:w202:T5, 3:w200:refnum<file>)  [unwired: 3 in, 1 out]
              n34 = case shown="Kein Fehler" w206 {
                selector: w206 -> [_ w209]
                tunnel: [TRUE _] -> w205
                tunnel: [errorcluster {"status"=FALSE, "code"=0, "source"=""} ("error IO") w209] -> w201
                frame No Error {
                }
                frame Error {
                  n35 = Wait (ms)(milliseconds to wait=u32 100 ("Zu wartende ms")) -> ()  [unwired: 1 out]
                }
              }
            }
            n36 = Close File(refnum=w194, error in=w196) -> (error out=w195:errorcluster)  [unwired: 1 out]
          }
        }
        n37 = Unbundle By Name(w158) -> ("Komponentenauswahl"=w160:T6)
        n38 = Empty Array?(array=w160) -> (empty?=w162:bool)
        n39 = Select(t=T6 [{"Komponente:"=0, "Konzentration"=0.0}, {"Komponente:"=0, "Konzentration"=0.0}, {"Komponente:"=0, "Konzentration"=0.0}, {"Komponente:"=0, "Konzentration"=0.0}, {"Komponente:"=0, "Konzentration"=0.0}, {"Komponente:"=0, "Konzentration"=0.0}] ("Wert (signalisierend)"), s=w162, f=w160) -> (s? t:f=w157:T6)
        n40 = Bundle By Name(cluster=w158, "Komponentenauswahl"=w157) -> (w159:T5)
        n41 = call <vilib>:"Clear Errors.vi"("error in (no error)"=w170) -> ()  [unwired: 5 in, 2 out]
      }
      frame "EPA auswerten" {
        n42 = Index Array(array=w226, index (dim 0)=w216) -> (element=w228:string[][])  [unwired: 2 in]
        n43 = Index Array(array=w218, index (col)=w216) -> (element=w217:bool[])  [unwired: 1 in]
        n44 = call "LinVer Protokoll_Daten.vi"("Lin-Polynom"=w227, "Aktiv"=w217, "Eingabetabelle"=w228) -> ("EPA Auswertung"=w223:cluster{sgl[], sgl[], bool[]}, "Ausgangs-Cluster"=w222:T5, "Tabelle"=w224:T4)  [unwired: 5 in, 1 out]
        n45 = Replace Array Subset(array=w226, new element=w224, index (dim 0)=w216) -> (w225:string[][][])  [unwired: 2 in]
      }
      frame "Tab init" {
        n46 = call "Konstanten zum Tabellen initialisieren.vi"() -> ("Anzahl Gaskomponenten"=w231:i32, "Anzahl Tabellenzeilen"=w232:i32, "Anzahl Tabellenspalten"=w233:i32)  [unwired: 13 in]
        n47 = Initialize Array(FALSE, w232, w231) -> (w239:bool[][])
        n48 = Initialize Array("----", w231, w232, w233) -> (w247:string[][][])
        n49 = Initialize Array("----", w231, w232, 3 ("Dimension")) -> (w243:string[][][])
        n50 = Initialize Array("----", 3 ("Dimension"), w231) -> (w235:string[][])
      }
      frame "Tab init ohne Stufen" {
        # "#TableStayFix"
        n51 = call "Konstanten zum Tabellen initialisieren.vi"() -> ("Anzahl Gaskomponenten"=w254:i32, "Anzahl Tabellenzeilen"=w255:i32, "Anzahl Tabellenspalten"=w256:i32)  [unwired: 13 in]
        n52 = Initialize Array(FALSE, w255, w254) -> (w259:bool[][])
        n53 = Initialize Array("----", w254, w255, w256) -> (w264:string[][][])
      }
      frame "Tabelle löschen" {
        n54 = call "Konstanten zum Tabellen initialisieren.vi"() -> ("Anzahl Gaskomponenten"=w271:i32, "Anzahl Tabellenzeilen"=w270:i32, "Anzahl Tabellenspalten"=w269:i32)  [unwired: 13 in]
        n55 = Initialize Array(FALSE, w270, w271) -> (w275:bool[][])
        n56 = Initialize Array("----", w271, w270, w269) -> (w281:string[][][])
      }
      frame "Stufentabelle" {
        n57 = Replace Array Subset(array=w296, new element="Stufen Tabelle", index (dim 0)=w294) -> (w295:string[][][])  [unwired: 2 in]
      }
      frame "EGAK Tab" {
        n58 = Replace Array Subset(array=w307, new element="EGAK", index (col)=w304) -> (w306:string[][])  [unwired: 1 in]
      }
      frame "EPA aktiviert" {
        n59 = Replace Array Subset(array=w325, new element=w322, index (col)=w323) -> (w324:bool[][])  [unwired: 1 in]
      }
      frame "LIN aktiviert" {
        n60 = Replace Array Subset(array=w338, new element=w340, index (col)=w339) -> (w337:bool[][])  [unwired: 1 in]
      }
      frame "Nachbehandlung laden" {
      }
      frame "Istwerte löschen" {
        n61 = for {
          tunnel: w368 -> [w377] mode=indexing
          tunnel: [w376] -> w367 mode=indexing
          # "Gasnr."
          n62 = for {
            tunnel: w377 -> [w379] mode=indexing
            tunnel: [w378] -> w376 mode=indexing
            # "Zeile"
            n63 = for {
              tunnel: w379 -> [w381] mode=indexing
              tunnel: [w380] -> w378 mode=indexing
              i -> [w383]
              # "Spalte"
              n64 = Equal To 0?(x=w383) -> (x = 0?=w382:bool)
              n65 = case shown="False" w382 {
                tunnel: w381 -> [_ w385]
                tunnel: ["----" w385] -> w380
                frame False {
                }
                frame True {
                }
              }
            }
          }
        }
      }
      frame "Zeile löschen" {
        n66 = Transpose 2D Array(2D array=w397) -> (transposed array=w396:bool[][])
        n67 = Transpose 2D Array(2D array=w392) -> (transposed array=w394:bool[][])
        n68 = for {
          tunnel: w396 -> [w411] mode=indexing
          tunnel: w390 -> [w412]
          tunnel: [w410] -> w398 mode=indexing
          n69 = Delete From Array(array=w411, index=w412) -> (array with subset deleted=w410:bool[])  [unwired: 1 in, 1 out]
        }
        n70 = for {
          tunnel: w394 -> [w409] mode=indexing
          tunnel: [w408] -> w393 mode=indexing
          tunnel: w390 -> [w407]
          n71 = Delete From Array(array=w409, index=w407) -> (array with subset deleted=w408:bool[])  [unwired: 1 in, 1 out]
        }
        n72 = for {
          tunnel: w400 -> [w416] mode=indexing
          tunnel: [w413] -> w399 mode=indexing
          tunnel: w390 -> [w415]
          # "Gasnr."
          n73 = for {
            tunnel: w416 -> [w418] mode=indexing
            tunnel: [w418] -> w414 mode=indexing if=w417
            tunnel: w415 -> [w420]
            i -> [w419]
            # "Zeile"
            n74 = Not Equal?(x=w419, y=w420) -> (x != y?=w417:bool)
          }
          n75 = call "Tabelle auffeullen.vi"("Neue Tabelle"=w414) -> ("Tabelle"=w413:string[][])  [unwired: 10 in]
        }
        n76 = Transpose 2D Array(2D array=w398) -> (transposed array=w395:bool[][])
        n77 = Transpose 2D Array(2D array=w393) -> (transposed array=w391:bool[][])
      }
      frame "Zeile einfügen" {
        n78 = Transpose 2D Array(2D array=w432) -> (transposed array=w431:bool[][])
        n79 = Transpose 2D Array(2D array=w427) -> (transposed array=w429:bool[][])
        n80 = for {
          tunnel: w435 -> [w453] mode=indexing
          tunnel: [w454] -> w434 mode=indexing
          tunnel: w425 -> [w452]
          # "Gasnr."
          n81 = Insert Into Array(array=w453, index (row)=w452, new element=string[] ["0"] ("Neues Element/Teil-Array")) -> (w451:string[][])  [unwired: 1 in]
          n82 = call "Tabelle auffeullen.vi"("Neue Tabelle"=w451) -> ("Tabelle"=w454:string[][])  [unwired: 10 in]
        }
        n83 = for {
          tunnel: w431 -> [w449] mode=indexing
          tunnel: w425 -> [w447]
          tunnel: [w446] -> w433 mode=indexing
          n84 = Insert Into Array(array=w449, index=w447, new element=TRUE ("Neues Element/Teil-Array")) -> (w446:bool[])
        }
        n85 = for {
          tunnel: w429 -> [w445] mode=indexing
          tunnel: w425 -> [w443]
          tunnel: [w442] -> w428 mode=indexing
          n86 = Insert Into Array(array=w445, index=w443, new element=TRUE ("Neues Element/Teil-Array")) -> (w442:bool[])
        }
        n87 = Transpose 2D Array(2D array=w433) -> (transposed array=w430:bool[][])
        n88 = Transpose 2D Array(2D array=w428) -> (transposed array=w426:bool[][])
      }
      frame "LIN/EPA aktiv laden" {
      }
    }
  }
  "Lin-Polynom" <- w6
  "Eingabetabelle" <- w11
  "EPA Auswertung" <- w10
  "Stufen Tabelle" <- w9
  "Aktiv EPA" <- w8
  "TabellenArray" <- w7
  "Aktiv LIN" <- w5
  "EKAG" <- w4
  "Ergebnis Lin" <- w3
  "Index (Seite) out" <- w2
  "error out" <- "error in (no error)"
